vi "Read Test Info.vi"(1 "Parameter Name Table":string[](array[string])) -> (0 "Parameter Table":string[][](array[string]))   [LabVIEW 2010]
uses:
  StateFile.llb/Actions.ctl
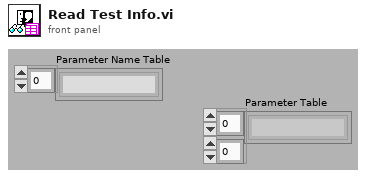
[diagram p1: front panel]
types:
  T1 = cluster{"Additional Parameter Section":string, "Blowfish Master Password":string, "Key Name":string, "Use Encryption":bool}
  T2 = typedef "Actions.ctl" = enum16{"Initialize", "Save VI State", "Load VI State", "Delete State", "Get All VI State Names", "Clear All States", "Close Global State File", "Open State File", "Create State File", "Write Data to File", "Exit"}
  T3 = typedef "Internal State Data.ctl" = cluster{"StateFile Reference":T4, "StateFile Filepath":path, "Error":errorcluster, "VI ":enum16{"By VI Name", "Calling VI"}, "VI Name":path, "State":enum16{"By State Name", "Default State"}, "State Name":string, "notifier in":refnum<notifier>, " Progress Bar":bool}
  T4 = typedef "NI_LVConfig.lvlib/Config Data RefNum.ctl" = refnum<k1>
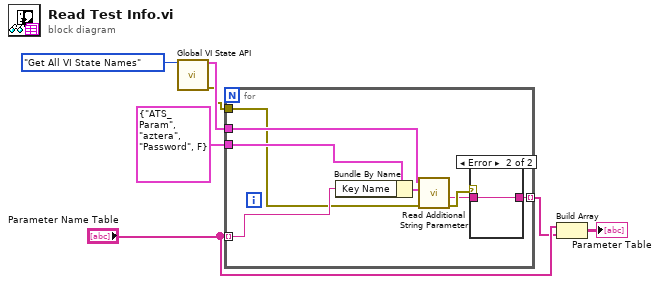
[diagram p0: block diagram]
diagram:
  n1 = call "Global VI State API.vi"("Action"=Actions."Get All VI State Names") -> ("Internal State Data"=w7:T3, "Error"=w1:errorcluster)  [unwired: 12 in, 1 out]
  n2 = for {
    tunnel: T1 {"Additional Parameter Section"="ATS_Param", "Blowfish Master Password"="aztera", "Key Name"="Password", "Use Encryption"=FALSE} ("Additional Parameters Out") -> [w15]
    tunnel: w7 -> [w14]
    tunnel: "Parameter Name Table" -> [w12] mode=indexing
    tunnel: [w8] -> w3 mode=indexing
    tunnel: w1 -> [w11]
    n3 = Bundle By Name(cluster=w15, "Key Name"=w12) -> (w13:T1)
    n4 = call "Read Additional String Parameter.vi"("error in (no error)"=w11, "Additional Parameters Out"=w13, "Internal State Data"=w14) -> ("error out"=w10:errorcluster, "Value"=w9:string)  [unwired: 5 in, 2 out]
    n5 = case shown="Error" w10 {
      tunnel: w9 -> [w16 w17]
      tunnel: [w16 w17] -> w8
      frame No Error {
      }
      frame Error {
      }
    }
  }
  n6 = Build Array("Parameter Name Table", w3) -> (→"Parameter Table":string[][])
